vi "AScan to Volts.vi"(8 "error in (no error)":errorcluster, 10 "A-Scan Number In":dbl, 11 "Galvo in":refnum<class "Galvo.lvclass">) -> (0 "error out":errorcluster, 2 "A-Scan in Volts":dbl, 3 "Galvo out":refnum<class "Galvo.lvclass">)   [LabVIEW 2015, in "Galvo.lvclass"]
uses:
  Galvo.lvclass
  Galvo.lvclass/Galvo.ctl
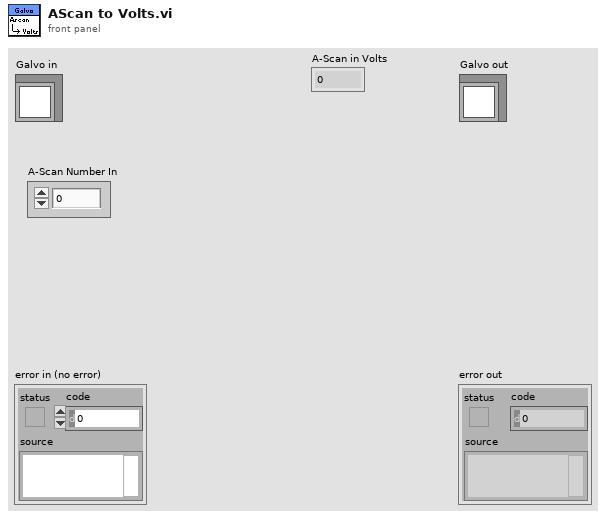
[diagram p1: front panel]
types:
  T1 = typedef "Galvo.lvclass/Fast Axis Parameters.ctl" = cluster{"Fast Axis Voltage":dbl, "Laser Sweep Frequency":dbl, "A-Scans in Fast Axis":dbl}
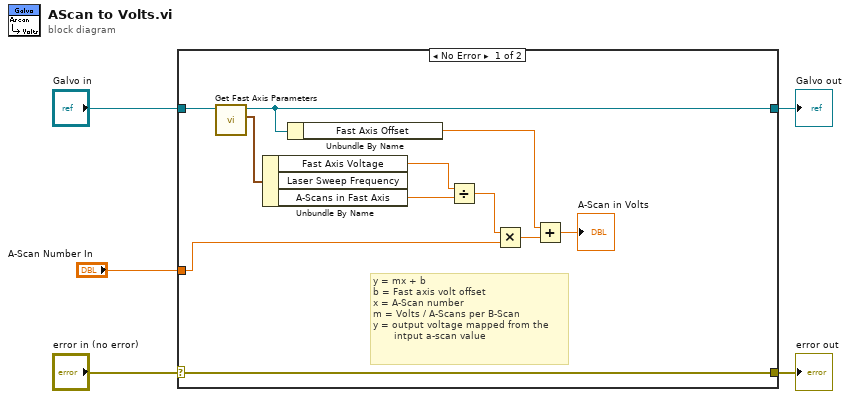
[diagram p0: block diagram]
diagram:
  n1 = case shown="No Error" "error in (no error)" {
    selector: "error in (no error)" -> [w16 w18]
    tunnel: [w16 w18] -> w4
    tunnel: [w11 w17] -> w2
    tunnel: "Galvo in" -> [w15 w17]
    tunnel: "A-Scan Number In" -> [w9 _]
    frame No Error {
      # "y = mx + b\nb = Fast axis volt offset\nx = A-Scan number\nm = Volts / A-Scans per B-Scan\ny = output voltage mapped from the\n       intput a-scan value"
      n2 = call-dynamic "Get Fast Axis Parameters.vi"("Galvo in"=w15) -> ("Fast Axis Parameters"=w14:T1, "Galvo out"=w11:refnum<class "Galvo.lvclass">)  [unwired: 8 in, 1 out]
      n3 = Unbundle By Name(w14) -> ("Fast Axis Voltage"=w13:dbl, "A-Scans in Fast Axis"=w12:dbl)  [unwired: 1 out]
      n4 = Unbundle By Name(w11) -> ("Fast Axis Offset"=w7:sgl)
      n5 = Divide(x=w13, y=w12) -> (x/y=w10:dbl)
      n6 = Multiply(x=w10, y=w9) -> (x*y=w8:dbl)
      n7 = Add(x=w7, y=w8) -> (x+y=→"A-Scan in Volts":dbl)
    }
    frame Error {
    }
  }
  "error out" <- w4
  "Galvo out" <- w2
